vi "PH_Switch_USB.PC _States.vi"(0 "i ref in":refnum<vi>, 1 "data":i8[](array[numeric]), 2 "serviceName":string, 3 "typeDescriptor":string, 4 "no link":bool, 5 "error IO":errorcluster) -> (14 "i ref out":refnum<vi>, 19 "error out":errorcluster)   [LabVIEW 2014, in "PH_Switch_USB.lvlib"]
doc: "This VI is the Proc Case \"_States\"; it writes incoming data to own attributes, calculates the device state and puts the information to the GUI."
uses:
  PH_Switch_USB.lvlib
  PH_Basics/PH_StatusHandler/PH_StatusHandler.Status.ctl
  PH_Basics/PH_Common/PH_Common.lvlib
  PH_Basics/PH_StatusHandler/PH_StatusHandler.lvlib
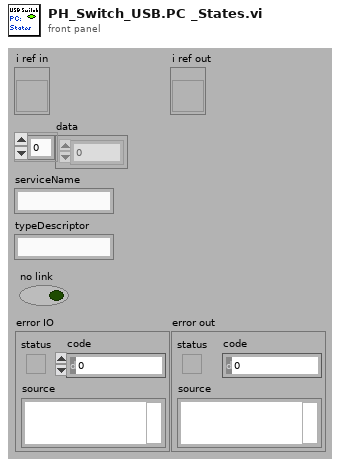
[diagram p1: front panel]
types:
  T1 = typedef "PH_Switch_USB.lvlib/PH_Switch_USB.i attribute.ctl" = cluster{"GUI Refs":cluster{"GUI-Knob":refnum<vi>, "Delete":refnum<vi>}, "Switch":cluster{"GUI Ref":refnum<vi>, "Service name":string, "Array No.":i16, "caption":string, "Status":T2}, "True-Sensor":cluster{"GUI Ref":refnum<vi>, "Service name":string, "Array No.":i16, "caption":string, "Status":T2}, "False-Sensor":cluster{"GUI Ref":refnum<vi>, "Service name":string, "Array No.":i16, "caption":string, "Status":T2}}
  T2 = typedef "PH_StatusHandler.lvlib/PH_StatusHandler.Status.ctl" = i16
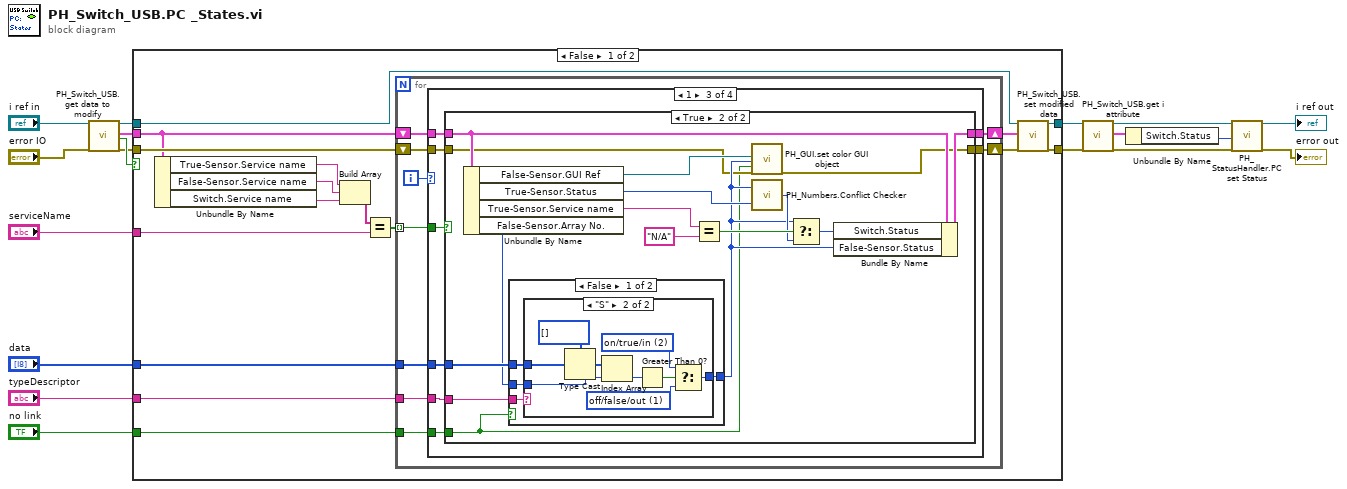
[diagram p0: block diagram]
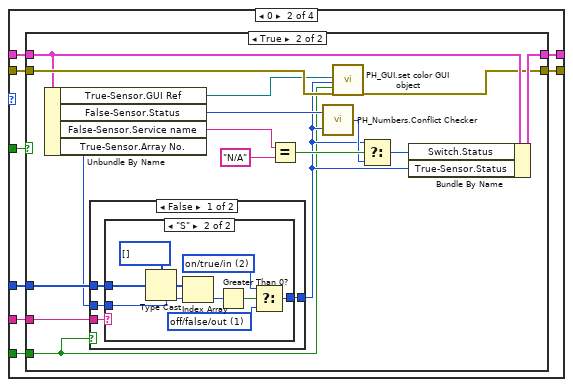
[diagram p3: hidden frame]
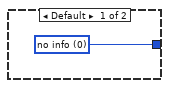
[diagram p5: hidden frame]
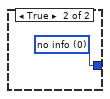
[diagram p6: hidden frame]
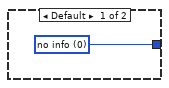
[diagram p8: hidden frame]
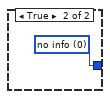
[diagram p9: hidden frame]
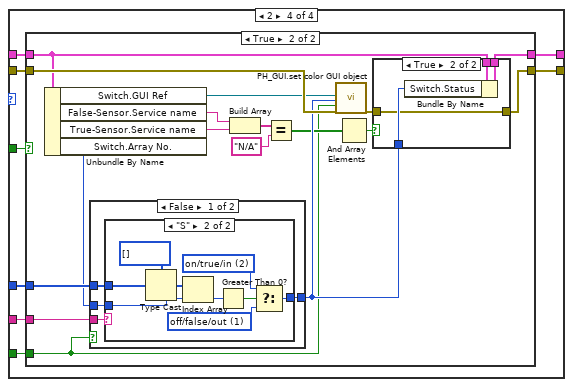
[diagram p10: hidden frame]
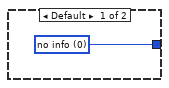
[diagram p13: hidden frame]
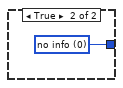
[diagram p14: hidden frame]
diagram:
  n1 = call "PH_Switch_USB.get data to modify.vi"("i ref in"="i ref in", "error in (no error)"="error IO") -> ("i ref out"=w16:refnum<vi>, "i attribute"=w17:T1, "timed out"=w18:bool, "error out"=w15:errorcluster)  [unwired: 14 in]
  n2 = case shown="False" w18 {
    tunnel: "typeDescriptor" -> [w30 _]
    tunnel: "data" -> [w29 _]
    tunnel: "no link" -> [w31 _]
    tunnel: w15 -> [w34 w177]
    tunnel: [w19 w177] -> w3
    tunnel: [w20 w176] -> w5
    tunnel: w16 -> [w24 w176]
    tunnel: w17 -> [w28 _]
    tunnel: "serviceName" -> [w22 _]
    frame False {
      n3 = Unbundle By Name(w28) -> ("True-Sensor.Service name"=w25:string, "False-Sensor.Service name"=w26:string, "Switch.Service name"=w27:string)
      n4 = Build Array(w25, w26, w27) -> (w23:string[])
      n5 = Equal?(x=w23, y=w22) -> (x = y?=w21:bool[])
      n6 = for {
        tunnel: w31 -> [w40]
        tunnel: w30 -> [w39]
        tunnel: w29 -> [w38]
        shift-right: [w41] -> w32
        shift-left: w28 -> [w37]
        shift-right: [w42] -> w33
        shift-left: w34 -> [w43]
        tunnel: w21 -> [w36] mode=indexing
        i -> [w35]
        n7 = case shown="1" w35 {
          tunnel: w43 -> [w44 w53 w94 w135]
          tunnel: [w44 w52 w93 w134] -> w42
          tunnel: [w45 w51 w92 w133] -> w41
          tunnel: w40 -> [_ w50 w91 w132]
          tunnel: w39 -> [_ w49 w90 w131]
          tunnel: w38 -> [_ w48 w89 w130]
          tunnel: w37 -> [w45 w47 w88 w129]
          tunnel: w36 -> [_ w46 w87 w128]
          frame Default {
          }
          frame 0 {
            n8 = case shown="True" w46 {
              tunnel: w53 -> [w54 w71]
              tunnel: [w54 w56] -> w52
              tunnel: [w55 w69] -> w51
              tunnel: w50 -> [_ w57]
              tunnel: w49 -> [_ w62]
              tunnel: w48 -> [_ w61]
              tunnel: w47 -> [w55 w59]
              frame False {
              }
              frame True {
                n9 = Unbundle By Name(w59) -> ("True-Sensor.GUI Ref"=w70:refnum<vi>, "False-Sensor.Status"=w66:T2, "False-Sensor.Service name"=w68:string, "True-Sensor.Array No."=w60:i16)
                n10 = case shown="False" w57 {
                  tunnel: [w74 w86] -> w63
                  tunnel: w62 -> [w75 _]
                  tunnel: w61 -> [w73 _]
                  tunnel: w60 -> [w72 _]
                  frame False {
                    n11 = case shown="\"S\"" w75 {
                      tunnel: [w76 w79] -> w74
                      tunnel: w73 -> [_ w84]
                      tunnel: w72 -> [_ w82]
                      frame Default {
                        w76 = T2 0 items=["no info", "off/false/out", "on/true/in", "Failure", "Alarm", "Status 1", "Status 2", "Status 3"] ("True-Sensor.Status")
                      }
                      frame "S" {
                        w77 = T2 1 items=["no info", "off/false/out", "on/true/in", "Failure", "Alarm", "Status 1", "Status 2", "Status 3"] ("True-Sensor.Status")
                        w78 = T2 2 items=["no info", "off/false/out", "on/true/in", "Failure", "Alarm", "Status 1", "Status 2", "Status 3"] ("True-Sensor.Status")
                        n12 = Type Cast(type=i16[] [], x=w84) -> (*(type *) &x=w83:i16[])
                        n13 = Index Array(array=w83, index=w82) -> (element=w81:i16)
                        n14 = Greater Than 0?(x=w81) -> (x > 0?=w80:bool)
                        n15 = Select(t=w78, s=w80, f=w77) -> (s? t:f=w79:T2)
                      }
                    }
                  }
                  frame True {
                    w86 = T2 0 items=["no info", "off/false/out", "on/true/in", "Failure", "Alarm", "Status 1", "Status 2", "Status 3"] ("True-Sensor.Status")
                  }
                }
                n16 = Equal?(x=w68, y="N/A" ("x")) -> (x = y?=w65:bool)
                n17 = call "PH_Numbers.Conflict Checker.vi"("Input 2"=w63, "Input 1"=w66) -> ("Result"=w64:i32)
                n18 = call "PH_GUI.set color GUI object.vi"("GUI object Ref"=w70, "State"=w63, "Blinking? (false)"=w57, "error in (no error)"=w71) -> ("error out"=w56:errorcluster)  [unwired: 15 in]
                n19 = Select(t=w63, s=w65, f=w64) -> (s? t:f=w58:i32)
                n20 = Bundle By Name(cluster=w59, "Switch.Status"=w58, "True-Sensor.Status"=w63) -> (w69:T1)
              }
            }
          }
          frame 1 {
            n21 = case shown="True" w87 {
              tunnel: w94 -> [w95 w99]
              tunnel: [w95 w97] -> w93
              tunnel: [w96 w111] -> w92
              tunnel: w91 -> [_ w98]
              tunnel: w90 -> [_ w106]
              tunnel: w89 -> [_ w105]
              tunnel: w88 -> [w96 w103]
              frame False {
              }
              frame True {
                n22 = Unbundle By Name(w103) -> ("False-Sensor.GUI Ref"=w112:refnum<vi>, "True-Sensor.Status"=w102:T2, "True-Sensor.Service name"=w110:string, "False-Sensor.Array No."=w104:i16)
                n23 = case shown="False" w98 {
                  tunnel: [w115 w127] -> w101
                  tunnel: w106 -> [w116 _]
                  tunnel: w105 -> [w114 _]
                  tunnel: w104 -> [w113 _]
                  frame False {
                    n24 = case shown="\"S\"" w116 {
                      tunnel: [w117 w120] -> w115
                      tunnel: w114 -> [_ w125]
                      tunnel: w113 -> [_ w123]
                      frame Default {
                        w117 = T2 0 items=["no info", "off/false/out", "on/true/in", "Failure", "Alarm", "Status 1", "Status 2", "Status 3"] ("True-Sensor.Status")
                      }
                      frame "S" {
                        w118 = T2 1 items=["no info", "off/false/out", "on/true/in", "Failure", "Alarm", "Status 1", "Status 2", "Status 3"] ("True-Sensor.Status")
                        w119 = T2 2 items=["no info", "off/false/out", "on/true/in", "Failure", "Alarm", "Status 1", "Status 2", "Status 3"] ("True-Sensor.Status")
                        n25 = Type Cast(type=i16[] [], x=w125) -> (*(type *) &x=w124:i16[])
                        n26 = Index Array(array=w124, index=w123) -> (element=w122:i16)
                        n27 = Greater Than 0?(x=w122) -> (x > 0?=w121:bool)
                        n28 = Select(t=w119, s=w121, f=w118) -> (s? t:f=w120:T2)
                      }
                    }
                  }
                  frame True {
                    w127 = T2 0 items=["no info", "off/false/out", "on/true/in", "Failure", "Alarm", "Status 1", "Status 2", "Status 3"] ("True-Sensor.Status")
                  }
                }
                n29 = Equal?(x=w110, y="N/A" ("x")) -> (x = y?=w108:bool)
                n30 = call "PH_GUI.set color GUI object.vi"("GUI object Ref"=w112, "State"=w101, "Blinking? (false)"=w98, "error in (no error)"=w99) -> ("error out"=w97:errorcluster)  [unwired: 15 in]
                n31 = call "PH_Numbers.Conflict Checker.vi"("Input 2"=w102, "Input 1"=w101) -> ("Result"=w107:i32)
                n32 = Select(t=w101, s=w108, f=w107) -> (s? t:f=w100:i32)
                n33 = Bundle By Name(cluster=w103, "Switch.Status"=w100, "False-Sensor.Status"=w101) -> (w111:T1)
              }
            }
          }
          frame 2 {
            n34 = case shown="True" w128 {
              tunnel: w135 -> [w136 w154]
              tunnel: [w136 w151] -> w134
              tunnel: [w137 w150] -> w133
              tunnel: w132 -> [_ w138]
              tunnel: w131 -> [_ w148]
              tunnel: w130 -> [_ w147]
              tunnel: w129 -> [w137 w145]
              frame False {
              }
              frame True {
                n35 = Unbundle By Name(w145) -> ("Switch.GUI Ref"=w153:refnum<vi>, "False-Sensor.Service name"=w142:string, "True-Sensor.Service name"=w143:string, "Switch.Array No."=w146:i16)
                n36 = case shown="False" w138 {
                  tunnel: [w163 w175] -> w144
                  tunnel: w148 -> [w164 _]
                  tunnel: w147 -> [w162 _]
                  tunnel: w146 -> [w161 _]
                  frame False {
                    n37 = case shown="\"S\"" w164 {
                      tunnel: [w165 w168] -> w163
                      tunnel: w162 -> [_ w173]
                      tunnel: w161 -> [_ w171]
                      frame Default {
                        w165 = T2 0 items=["no info", "off/false/out", "on/true/in", "Failure", "Alarm", "Status 1", "Status 2", "Status 3"] ("True-Sensor.Status")
                      }
                      frame "S" {
                        w166 = T2 1 items=["no info", "off/false/out", "on/true/in", "Failure", "Alarm", "Status 1", "Status 2", "Status 3"] ("True-Sensor.Status")
                        w167 = T2 2 items=["no info", "off/false/out", "on/true/in", "Failure", "Alarm", "Status 1", "Status 2", "Status 3"] ("True-Sensor.Status")
                        n38 = Type Cast(type=i16[] [], x=w173) -> (*(type *) &x=w172:i16[])
                        n39 = Index Array(array=w172, index=w171) -> (element=w170:i16)
                        n40 = Greater Than 0?(x=w170) -> (x > 0?=w169:bool)
                        n41 = Select(t=w167, s=w169, f=w166) -> (s? t:f=w168:T2)
                      }
                    }
                  }
                  frame True {
                    w175 = T2 0 items=["no info", "off/false/out", "on/true/in", "Failure", "Alarm", "Status 1", "Status 2", "Status 3"] ("True-Sensor.Status")
                  }
                }
                n42 = Build Array(w142, w143) -> (w141:string[])
                n43 = Equal?(x=w141, y="N/A" ("x")) -> (x = y?=w140:bool[])
                n44 = call "PH_GUI.set color GUI object.vi"("GUI object Ref"=w153, "State"=w144, "Blinking? (false)"=w138, "error in (no error)"=w154) -> ("error out"=w152:errorcluster)  [unwired: 15 in]
                n45 = And Array Elements(Boolean array=w140) -> (logical AND=w139:bool)
                n46 = case shown="True" w139 {
                  tunnel: w152 -> [w155 w157]
                  tunnel: [w155 w157] -> w151
                  tunnel: [w156 w160] -> w150
                  tunnel: w145 -> [w156 w159]
                  tunnel: w144 -> [_ w158]
                  frame False {
                  }
                  frame True {
                    n47 = Bundle By Name(cluster=w159, "Switch.Status"=w158) -> (w160:T1)
                  }
                }
              }
            }
          }
        }
      }
      n48 = call "PH_Switch_USB.set modified data.vi"("i ref in"=w24, "i attribute"=w32, "error in (no error)"=w33) -> ("i ref out"=w20:refnum<vi>, "error out"=w19:errorcluster)  [unwired: 15 in]
    }
    frame True {
    }
  }
  n49 = call "PH_Switch_USB.get i attribute.vi"("i ref in"=w5, "error in (no error)"=w3) -> ("i ref out"=w6:refnum<vi>, "i attribute"=w2:T1, "error out"=w4:errorcluster)  [unwired: 15 in]
  n50 = Unbundle By Name(w2) -> ("Switch.Status"=w1:T2)
  n51 = call "PH_StatusHandler.PC set Status.vi"("i ref in"=w6, "Status"=w1, "error in (no error)"=w4) -> ("i ref out"=→"i ref out":refnum<vi>, "error out"=→"error out":errorcluster)  [unwired: 15 in]
